vi "set PG according to private data.vi"(8 "error in (no error)":errorcluster, 11 "Pulse Gen Scan in":refnum<class "Pulse Gen Scan.lvclass">) -> (0 "error out":errorcluster, 3 "Pulse Gen Scan out":refnum<class "Pulse Gen Scan.lvclass">)   [LabVIEW 2009, in "Pulse Gen Scan.lvclass"]
uses:
  Pulse Gen Scan.lvclass
  Pulse Gen Scan.lvclass/Pulse Gen Scan.ctl
  Instruments/Utility Classes/Scannable/Scannable.lvclass
panel:
  out "Outputs on/off":bool[](array[boolean])
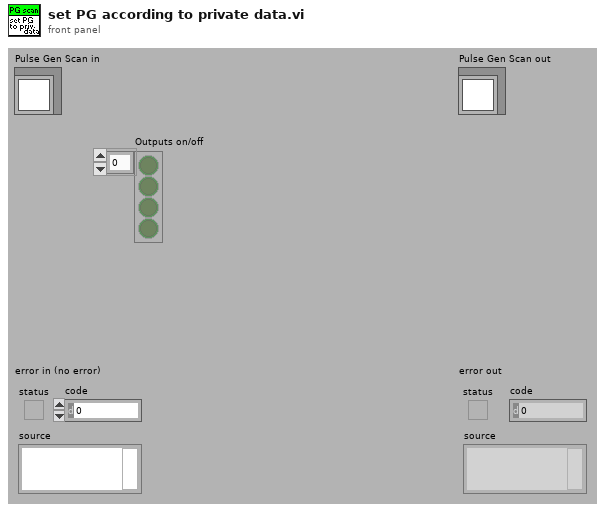
[diagram p1: front panel]
types:
  T1 = enum16{"Channel All ", "Channel 1", "Channel 2", "Channel 3", "Channels Combined"}
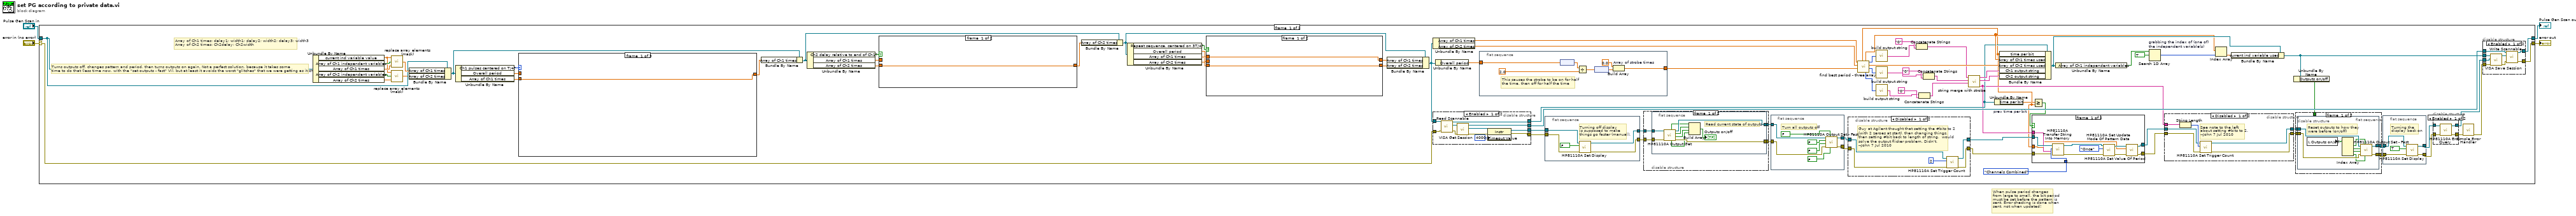
[diagram p0: block diagram]
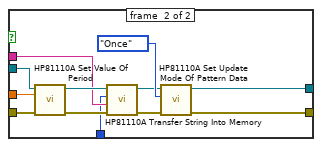
[diagram p2: hidden frame]
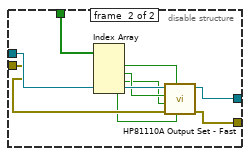
[diagram p3: hidden frame]
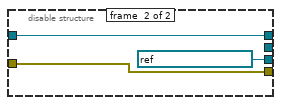
[diagram p6: hidden frame]
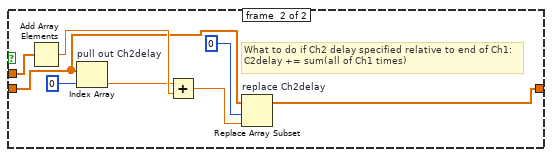
[diagram p10: hidden frame]
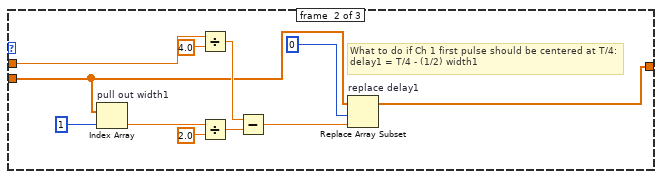
[diagram p11: hidden frame]
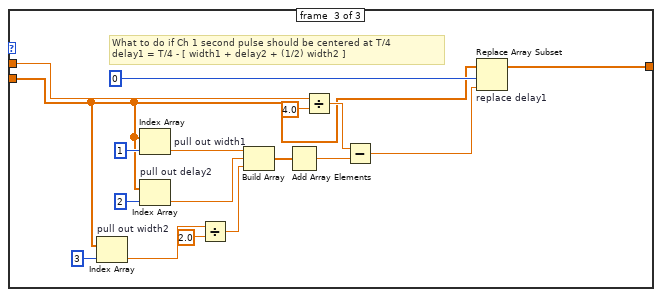
[diagram p12: hidden frame]
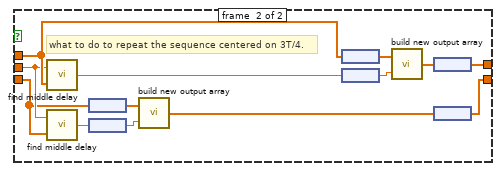
[diagram p13: hidden frame]
diagram:
  # "When pulse period changes\nfrom large to small, the bit period\nmust be set before the pattern is \nsent. Error checking is done when\nsent, not when updated!"
  n1 = case shown="No Error" "error in (no error)" {
    selector: "error in (no error)" -> [w53 w273]
    tunnel: [w49 w273] -> w3
    tunnel: "Pulse Gen Scan in" -> [w75 w272]
    tunnel: [w48 w272] -> w1
    frame #0 {
      # "Turns outputs off, changes pattern and period, then turns outputs on again. Not a perfect solution, because it takes some \ntime to do that (less time now, with the \"set outputs - fast\" VI), but at least it avoids the worst \"glitches\" that we were getting as it changed pts."
      # "Array of Ch1 times: delay1; width1; delay2; width2; delay3; width3\nArray of Ch2 times: Ch2delay; Ch2width"
      n2 = Unbundle By Name(w75) -> ("current ind variable value"=w74:dbl[unit], "Array of Ch1 independent variables"=w80:bool[], "Array of Ch1 times"=w79:dbl[unit][], "Array of Ch2 independent variables"=w73:bool[], "Array of Ch2 times"=w72:dbl[unit][])
      n3 = call "replace array elements (mask).vi"("input array of numbers"=w79, "array of booleans (mask)"=w80, "value"=w74) -> ("output array"=w76:dbl[unit][])
      n4 = call "replace array elements (mask).vi"("input array of numbers"=w72, "array of booleans (mask)"=w73, "value"=w74) -> ("output array"=w71:dbl[unit][])
      n5 = Bundle By Name(cluster=w75, "Array of Ch1 times"=w76, "Array of Ch2 times"=w71) -> (w69:refnum<class "Pulse Gen Scan.lvclass">)
      n6 = Unbundle By Name(w69) -> ("Ch1 pulses centered on T/4?"=w85:enum32{"none", "first", "second"}, "Overall period"=w78:dbl[unit], "Array of Ch1 times"=w77:dbl[unit][])
      n7 = case shown="\"second\"" w85 {
        tunnel: w77 -> [w228 w230 w242]
        tunnel: [w228 w232 w248] -> w70
        tunnel: w78 -> [_ w233 w249]
        frame #0 {
        }
        frame #1 {
          # "What to do if Ch 1 first pulse should be centered at T/4:\ndelay1 = T/4 - (1/2) width1"
          n8 = Index Array "pull out width1"(array=w230, index=1) -> (element=w229:dbl[unit])
          n9 = Divide(x=w233, y=4.0) -> (x/y=w238:dbl[unit])
          n10 = Divide(x=w229, y=2.0) -> (x/y=w236:dbl[unit])
          n11 = Subtract(x=w238, y=w236) -> (x-y=w234:dbl[unit])
          n12 = Replace Array Subset "replace delay1"(array=w230, new element=w234, index=0) -> (w232:dbl[unit][])
        }
        frame #2 {
          # "What to do if Ch 1 second pulse should be centered at T/4\ndelay1 = T/4 - [ width1 + delay2 + (1/2) width2 ]"
          n13 = Index Array "pull out width2"(array=w242, index=3) -> (element=w241:dbl[unit])
          n14 = Index Array "pull out width1"(array=w242, index=1) -> (element=w246:dbl[unit])
          n15 = Index Array "pull out delay2"(array=w242, index=2) -> (element=w244:dbl[unit])
          n16 = Divide(x=w241, y=2.0) -> (x/y=w251:dbl[unit])
          n17 = Build Array(w246, w244, w251) -> (w253:dbl[unit][])
          n18 = Add Array Elements(numeric array=w253) -> (sum=w252:dbl[unit])
          n19 = Divide(x=w249, y=4.0) -> (x/y=w255:dbl[unit])
          n20 = Subtract(x=w255, y=w252) -> (x-y=w240:dbl[unit])
          n21 = Replace Array Subset "replace delay1"(array=w242, new element=w240, index=0) -> (w248:dbl[unit][])
        }
      }
      n22 = Bundle By Name(cluster=w69, "Array of Ch1 times"=w70) -> (w54:refnum<class "Pulse Gen Scan.lvclass">)
      n23 = Unbundle By Name(w54) -> ("Ch2 delay relative to end of Ch1?"=w64:bool, "Array of Ch1 times"=w68:dbl[unit][], "Array of Ch2 times"=w63:dbl[unit][])
      n24 = case shown="True" w64 {
        tunnel: [w219 w222] -> w67
        tunnel: w63 -> [w219 w220]
        tunnel: w68 -> [_ w226]
        frame #0 {
        }
        frame #1 {
          # "What to do if Ch2 delay specified relative to end of Ch1:\nC2delay += sum(all of Ch1 times)"
          n25 = Add Array Elements(numeric array=w226) -> (sum=w227:dbl[unit])
          n26 = Index Array "pull out Ch2delay"(array=w220, index=0) -> (element=w221:dbl[unit])
          n27 = Add(x=w221, y=w227) -> (x+y=w223:dbl[unit])
          n28 = Replace Array Subset "replace Ch2delay"(array=w220, new element=w223, index=0) -> (w222:dbl[unit][])
        }
      }
      n29 = Bundle By Name(cluster=w54, "Array of Ch2 times"=w67) -> (w60:refnum<class "Pulse Gen Scan.lvclass">)
      n30 = Unbundle By Name(w60) -> ("Repeat sequence, centered on 3T/4?"=w61:bool, "Overall period"=w62:dbl[unit], "Array of Ch1 times"=w65:dbl[unit][], "Array of Ch2 times"=w66:dbl[unit][])
      n31 = case shown="True" w61 {
        tunnel: w65 -> [w258 w265]
        tunnel: [w258 w268] -> w59
        tunnel: w66 -> [w257 w260]
        tunnel: [w257 w266] -> w58
        tunnel: w62 -> [_ w263]
        frame #0 {
        }
        frame #1 {
          # "what to do to repeat the sequence centered on 3T/4."
          n32 = call "find middle delay.vi"("array of times"=w265, "Expected overall period"=w263) -> ("middle delay"=w264:dbl[unit])
          n33 = call "find middle delay.vi"("array of times"=w260, "Expected overall period"=w263) -> ("middle delay"=w262:dbl[unit])
          n34 = node(w260) -> (w259:dbl[])
          n35 = node(w262) -> (w261:dbl)
          n36 = call "build new output array.vi"("number to insert"=w261, "input array"=w259) -> ("output array"=w267:dbl[])
          n37 = node(w265) -> (w271:dbl[])
          n38 = node(w264) -> (w270:dbl)
          n39 = call "build new output array.vi"("number to insert"=w270, "input array"=w271) -> ("output array"=w269:dbl[])
          n40 = node(w269) -> (w268:dbl[unit][])
          n41 = node(w267) -> (w266:dbl[unit][])
        }
      }
      n42 = Bundle By Name(cluster=w60, "Array of Ch1 times"=w59, "Array of Ch2 times"=w58) -> (w25:refnum<class "Pulse Gen Scan.lvclass">)
      n43 = Unbundle By Name(w25) -> ("Array of Ch1 times"=w33:dbl[unit][], "Array of Ch2 times"=w32:dbl[unit][])
      n44 = disable-structure shown="Enabled" {
        disable-tunnel: w53 -> [w175 w179]
        disable-tunnel: [w174 w180] -> w12
        disable-tunnel: w25 -> [w173 w180]
        disable-tunnel: [w172 _] -> w51
        disable-tunnel: [w169 refnum<visa-resource-name> "GPIB0::10::INSTR" ("VISA Resource Name")] -> w47
        disable-tunnel: [w167 w179] -> w45
        frame #0 {
          n45 = call-dynamic "Read Scannable.vi"("error in (no error)"=w175, "Scanner.lvclass in"=w173) -> ("error out"=w176:errorcluster, "Scannable.lvclass"=w177:refnum<class "Scannable.lvclass">, "Scanner.lvclass out"=w174:refnum<class "Pulse Gen Scan.lvclass">)  [unwired: 7 out]
          n46 = call-dynamic "VISA Get Session.vi"("error in (no error)"=w176, "Instrument.lvclass in"=w177) -> ("error out"=w168:errorcluster, "VISA Resource Name"=w170:refnum<visa-resource-name>, "Instrument.lvclass out"=w172:refnum<class "Scannable.lvclass">)  [unwired: 7 out]
          n47 = property class="Instr"(reference=w170, error in=w168, "General Settings:Timeout Value"=u32 4000) -> (reference out=w169:refnum<visa-resource-name>, error out=w167:errorcluster)
        }
        frame #1 {
        }
      }
      n48 = Unbundle By Name(w25) -> ("Overall period"=w24:dbl[unit])
      n49 = flat-sequence {
        tunnel: [w153] -> w31
        tunnel: w24 -> [w152]
        frame #0 {
          # "This causes the strobe to be on for half the time, then off for half the time"
          n50 = node(w152) -> (w156:dbl)
          n51 = Divide(x=w156, y=2.0) -> (x/y=w154:dbl)
          n52 = node(w154) -> (w151:dbl[unit])
          n53 = Build Array "Array of strobe times"(dbl[unit] 0.0 ("element"), w151) -> (w153:dbl[unit][])
        }
      }
      n54 = flat-sequence {
        tunnel: w47 -> [w189]
        tunnel: [w188] -> w46
        tunnel: w45 -> [w187]
        tunnel: [w186] -> w44
        frame #0 {
          # "Turning off display\nis supposed to make \nthings go faster (manual)."
          n55 = call "HP81110A Set Display.vi"("error in (no error)"=w187, "Display (F:Off)"=FALSE, "VISA session"=w189) -> ("error out"=w186:errorcluster, "dup VISA session"=w188:refnum<visa-resource-name>)  [unwired: 7 out]
        }
      }
      n56 = disable-structure shown="Enabled" {
        disable-tunnel: [w138 w149] -> w82
        disable-tunnel: [w137 w148] -> w81
        disable-tunnel: w46 -> [w136 w149]
        disable-tunnel: w44 -> [w135 w148]
        frame #0 {
          n57 = flat-sequence {
            tunnel: [w147] -> w138
            tunnel: [w146] -> w137
            tunnel: w135 -> [w145]
            tunnel: w136 -> [w144]
            frame #0 {
              # "Read current state of outputs"
              n58 = call "HP81110A Output Get.vi"("error in (no error)"=w145, "VISA session"=w144) -> ("error out"=w146:errorcluster, "output2OUT"=w141:bool, "notoutput1OUT"=w142:bool, "dup VISA session"=w147:refnum<visa-resource-name>, "notoutput2OUT"=w140:bool, "output1OUT"=w143:bool)  [unwired: 4 out]
              n59 = Build Array(w143, w142, w141, w140) -> (→"Outputs on/off":bool[])
            }
          }
        }
        frame #1 {
        }
      }
      n60 = flat-sequence {
        tunnel: w82 -> [w198]
        tunnel: w81 -> [w197]
        tunnel: [w196] -> w43
        tunnel: [w195] -> w42
        frame #0 {
          # "Turn all outputs off"
          n61 = call "HP81110A Output Set - Fast.vi"("notoutput2"=FALSE, "output1"=FALSE, "error in (no error)"=w197, "output2"=FALSE, "notoutput1"=FALSE, "VISA session"=w198) -> ("error out"=w195:errorcluster, "dup VISA session"=w196:refnum<visa-resource-name>)  [unwired: 4 out]
        }
      }
      n62 = disable-structure shown="Disabled" {
        disable-tunnel: w43 -> [w210 w213]
        disable-tunnel: w42 -> [w209 w212]
        disable-tunnel: [w208 w212] -> w9
        disable-tunnel: [w207 w213] -> w10
        frame #0 {
          # "Guy at Agilent thought that setting the #bits to 2 \n(with 2 zeroes at start), then changing things, \nthen setting #bit back to length of string,  would \nsolve the output flicker problem. Didn't.\n--John 7 Jul 2010"
          n63 = call "HP81110A Set Trigger Count.vi"("error in (no error)"=w209, "Trigger Count"=2, "VISA session"=w210) -> ("error out"=w208:errorcluster, "dup VISA session"=w207:refnum<visa-resource-name>)  [unwired: 7 out]
        }
        frame #1 {
        }
      }
      n64 = call "find best period - three array.vi"("Array of strobe desired times"=w31, "Array of Ch2 desired times"=w32, "Array of Ch1 desired times"=w33) -> ("Array of Ch2 \"period-units\""=w27:i32[], "Array of Ch2 actual times"=w28:dbl[unit][], "Array of Ch1 \"period-units\""=w29:i32[], "Array of strobe \"period-units\""=w26:i32[], "Array of Ch1 actual times"=w30:dbl[unit][], "best period"=w5:dbl[unit])  [unwired: 2 in, 1 out]
      n65 = call "build output string.vi"("Array of \"period-units\""=w29) -> ("output string"=w20:string)
      n66 = call "build output string.vi"("Array of \"period-units\""=w27) -> ("output string"=w19:string)
      n67 = call "build output string.vi"("Array of \"period-units\""=w26) -> ("output string"=w18:string)
      n68 = Concatenate Strings(w20, "0" ("string")) -> (w17:string)
      n69 = Concatenate Strings(w18, "0" ("string")) -> (w15:string)
      n70 = Concatenate Strings(w19, "0" ("string")) -> (w16:string)
      n71 = call "string merge with strobe.vi"("Strobe String"=w15, "Ch2 String"=w16, "Ch1 String"=w17) -> ("Merged Output String"=w11:string, "Ch2 Output String"=w55:string, "Ch1 Output String"=w56:string)  [unwired: 5 in, 1 out]
      n72 = Unbundle By Name "prev time per bit"(w12) -> ("time per bit"=w7:dbl[unit])
      n73 = Bundle By Name(cluster=w12, "time per bit"=w5, "Array of Ch1 times used"=w30, "Array of Ch2 times used"=w28, "Ch1 output string"=w56, "Ch2 output string"=w55) -> (w57:refnum<class "Pulse Gen Scan.lvclass">)
      n74 = Greater Or Equal?(x=w7, y=w5) -> (x >= y?=w6:bool)
      n75 = case shown="True" w6 {
        tunnel: [w98 w110] -> w41
        tunnel: [w96 w111] -> w40
        tunnel: w11 -> [w92 w107]
        tunnel: w10 -> [w95 w104]
        tunnel: w9 -> [w93 w103]
        tunnel: T1."Channels Combined" ("Channel (1:Channel 1)") -> [w94 w102]
        tunnel: w5 -> [w89 w101]
        frame #0 {
          n76 = call "HP81110A Transfer String Into Memory.vi"("error in (no error)"=w93, "String"=w92, "Channel (1:Channel 1)"=w94, "VISA session"=w95) -> ("error out"=w90:errorcluster, "dup VISA session"=w91:refnum<visa-resource-name>)  [unwired: 6 out]
          n77 = call "HP81110A Set Update Mode Of Pattern Data.vi"("error in (no error)"=w90, "Pattern Update Mode (1:Continuous)"=enum16{"Off", "Continuous", "Once"}."Once", "VISA session"=w91) -> ("error out"=w97:errorcluster, "dup VISA session"=w99:refnum<visa-resource-name>)  [unwired: 7 out]
          n78 = call "HP81110A Set Value Of Period.vi"("error in (no error)"=w97, "Period Value"=w89, "VISA session"=w99) -> ("error out"=w96:errorcluster, "dup VISA session"=w98:refnum<visa-resource-name>)  [unwired: 7 out]
        }
        frame #1 {
          n79 = call "HP81110A Set Value Of Period.vi"("error in (no error)"=w103, "Period Value"=w101, "VISA session"=w104) -> ("error out"=w108:errorcluster, "dup VISA session"=w109:refnum<visa-resource-name>)  [unwired: 7 out]
          n80 = call "HP81110A Transfer String Into Memory.vi"("error in (no error)"=w108, "String"=w107, "Channel (1:Channel 1)"=w102, "VISA session"=w109) -> ("error out"=w105:errorcluster, "dup VISA session"=w106:refnum<visa-resource-name>)  [unwired: 6 out]
          n81 = call "HP81110A Set Update Mode Of Pattern Data.vi"("error in (no error)"=w105, "Pattern Update Mode (1:Continuous)"=enum16{"Off", "Continuous", "Once"}."Once", "VISA session"=w106) -> ("error out"=w111:errorcluster, "dup VISA session"=w110:refnum<visa-resource-name>)  [unwired: 7 out]
        }
      }
      n82 = Unbundle By Name(w57) -> ("Array of Ch1 independent variables"=w87:bool[])
      n83 = Search 1D Array "grabbing the index of (one of) \nthe independent variable(s)"(1D array=w87, element=TRUE) -> (index of element=w86:i32)  [unwired: 1 out]
      n84 = disable-structure shown="Disabled" {
        disable-tunnel: [w203 w206] -> w35
        disable-tunnel: [w202 w205] -> w34
        disable-tunnel: w41 -> [w201 w206]
        disable-tunnel: w40 -> [w200 w205]
        disable-tunnel: w11 -> [w199 _]
        frame #0 {
          # "See note to the left \nabout setting #bits to 2.\n--John 7 Jul 2010"
          n85 = String Length(string=w199) -> (length=w204:i32)
          n86 = call "HP81110A Set Trigger Count.vi"("error in (no error)"=w200, "Trigger Count"=w204, "VISA session"=w201) -> ("error out"=w202:errorcluster, "dup VISA session"=w203:refnum<visa-resource-name>)  [unwired: 7 out]
        }
        frame #1 {
        }
      }
      n87 = Index Array(array=w30, index=w86) -> (element=w84:dbl[unit])
      n88 = Bundle By Name(cluster=w57, "current ind variable used"=w84) -> (w14:refnum<class "Pulse Gen Scan.lvclass">)
      n89 = Unbundle By Name(w14) -> ("Outputs on/off"=w13:bool[])
      n90 = disable-structure shown="Enabled" {
        disable-tunnel: [w116 w131] -> w38
        disable-tunnel: [w115 w132] -> w36
        disable-tunnel: w35 -> [w114 w134]
        disable-tunnel: w34 -> [w113 w133]
        disable-tunnel: w13 -> [_ w130]
        frame #0 {
          n91 = flat-sequence {
            tunnel: [w125] -> w116
            tunnel: [w124] -> w115
            tunnel: w114 -> [w123]
            tunnel: w113 -> [w122]
            frame #0 {
              # "Reset outputs to how they \nwere before (on/off)"
              n92 = local read "Outputs on/off"() -> (w121:bool[])
              n93 = Index Array(array=w121) -> (element #1=w120:bool, element #2=w119:bool, element #3=w118:bool, element #4=w117:bool)  [unwired: 4 in]
              n94 = call "HP81110A Output Set - Fast.vi"("notoutput2"=w117, "output1"=w120, "error in (no error)"=w122, "output2"=w118, "notoutput1"=w119, "VISA session"=w123) -> ("error out"=w124:errorcluster, "dup VISA session"=w125:refnum<visa-resource-name>)  [unwired: 4 out]
            }
          }
        }
        frame #1 {
          n95 = Index Array(array=w130) -> (element #1=w129:bool, element #2=w128:bool, element #3=w127:bool, element #4=w126:bool)  [unwired: 4 in]
          n96 = call "HP81110A Output Set - Fast.vi"("notoutput2"=w126, "output1"=w129, "error in (no error)"=w133, "output2"=w127, "notoutput1"=w128, "VISA session"=w134) -> ("error out"=w132:errorcluster, "dup VISA session"=w131:refnum<visa-resource-name>)  [unwired: 4 out]
        }
      }
      n97 = flat-sequence {
        tunnel: [w184] -> w39
        tunnel: w38 -> [w183]
        tunnel: [w182] -> w37
        tunnel: w36 -> [w181]
        frame #0 {
          # "Turning the \ndisplay back on"
          n98 = call "HP81110A Set Display.vi"("error in (no error)"=w181, "Display (F:Off)"=TRUE, "VISA session"=w183) -> ("error out"=w182:errorcluster, "dup VISA session"=w184:refnum<visa-resource-name>)  [unwired: 7 out]
        }
      }
      n99 = disable-structure shown="Enabled" {
        disable-tunnel: [w217 w218] -> w83
        disable-tunnel: w39 -> [w216 _]
        disable-tunnel: w37 -> [w215 w218]
        disable-tunnel: [w214 _] -> w52
        frame #0 {
          n100 = call "HP81110A Error Query.vi"("VISA session"=w216, "error in (no error)"=w215) -> ("dup VISA session"=w214:refnum<visa-resource-name>, "error out"=w217:errorcluster)  [unwired: 12 out]
        }
        frame #1 {
        }
      }
      n101 = call <vilib>:"Simple Error Handler.vi"("error in (no error)"=w83) -> ("error out"=w50:errorcluster)  [unwired: 1 in, 7 out]
      n102 = disable-structure shown="Enabled" {
        disable-tunnel: w52 -> [w164 _]
        disable-tunnel: w51 -> [w163 _]
        disable-tunnel: w50 -> [w161 w165]
        disable-tunnel: [w160 w165] -> w49
        disable-tunnel: w14 -> [w159 w166]
        disable-tunnel: [w158 w166] -> w48
        frame #0 {
          n103 = call-dynamic "VISA Save Session.vi"("error in (no error)"=w161, "VISA Resource Name"=w164, "Instrument.lvclass in"=w163) -> ("error out"=w162:errorcluster, "Instrument.lvclass out"=w157:refnum<class "Scannable.lvclass">)  [unwired: 7 out]
          n104 = call-dynamic "Write Scannable.vi"("error in (no error)"=w162, "Scannable.lvclass"=w157, "Scanner.lvclass in"=w159) -> ("error out"=w160:errorcluster, "Scanner.lvclass out"=w158:refnum<class "Pulse Gen Scan.lvclass">)  [unwired: 7 out]
        }
        frame #1 {
        }
      }
    }
    frame #1 {
    }
  }
  "error out" <- w3
  "Pulse Gen Scan out" <- w1
